vi "AllTempToCalTubeTemp.vi"(11 "All Temps":dbl[](array[numeric])) -> (3 "Cal Tube Temps":dbl)   [LabVIEW 2018, in "Analysis.lvlib"]
uses:
  Analysis.lvlib
  <vilib>/Analysis/baseanly.llb/Mean (DBL).vi
  <vilib>/Analysis/NI_AALBase.lvlib
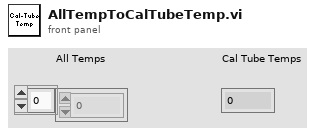
[diagram p1: front panel]
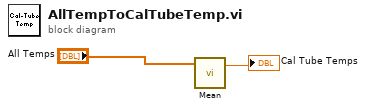
[diagram p0: block diagram]
diagram:
  n1 = call-poly <vilib>:"Mean.vi"("X"="All Temps") -> ("mean"=→"Cal Tube Temps":dbl)  [unwired: 1 out]
